vi "Receive_FocusRangeCm.vi"(3 "error in (no error)":errorcluster, 4 "Image mode":string(combo), 5 "Timeout (ms)":i32=40000000, 6 "connection ID in":refnum<k5>) -> (0 "error out":errorcluster, 1 "FocusRangeCm":dbl, 2 "connection ID out":refnum<k5>)   [LabVIEW 2016]
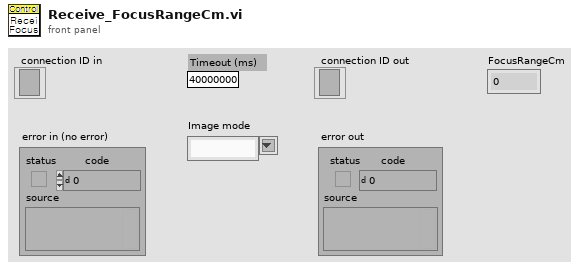
[diagram p1: front panel]
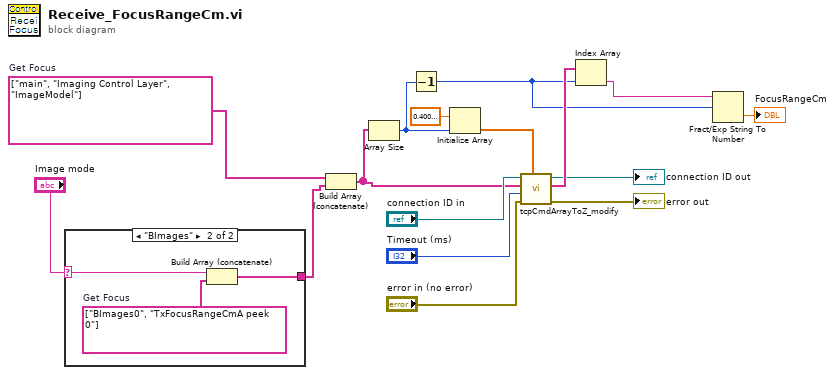
[diagram p0: block diagram]
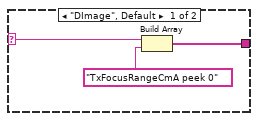
[diagram p2: hidden frame]
diagram:
  w6 = string[] ["main", "Imaging Control Layer", "ImageModel"]  # Get Focus
  n1 = case shown="\"BImages\"" "Image mode" {
    selector: "Image mode" -> [w19 w22]
    tunnel: [w17 w20] -> w2
    frame "DImage", Default {
      n2 = Build Array(w19, "TxFocusRangeCmA peek 0") -> (w17:string[])
    }
    frame "BImages" {
      w21 = string[] ["BImages0", "TxFocusRangeCmA peek 0"]  # Get Focus
      n3 = Build Array (concatenate)(w22, w21) -> (w20:string[])
    }
  }
  n4 = Build Array (concatenate)(w6, w2) -> (w5:string[])
  n5 = Array Size(array=w5) -> (size(s)=w13:i32)
  n6 = Decrement(x=w13) -> (x-1=w1:i32)
  n7 = Initialize Array(sgl 0.4 ("element"), w13) -> (w15:sgl[])
  n8 = call "tcpCmdArrayToZ_modify.vi"("Delay (sec)"=w15, "error in (no error)"="error in (no error)", "Timeout (ms)"="Timeout (ms)", "Command array"=w5, "connection ID in"="connection ID in") -> ("error out"=→"error out":errorcluster, "Receive array"=w14:string[], "connection ID out"=→"connection ID out":refnum<k5>)  [unwired: 2 in, 2 out]
  n9 = Index Array(array=w14, index=w1) -> (element=w3:string)
  n10 = Fract/Exp String To Number(string=w3, offset=w1) -> (number=→"FocusRangeCm":dbl)  [unwired: 2 in, 1 out]
